vi "Main.vi"() -> ()   [LabVIEW 2021]
panel:
  in  "Numeric":u64 format="%x"
  out "substring":string
  in  "dato":string="F039"
  in  "Write":bool
  in  "Read":bool
  in  "stop":bool
  out "CompleteFrame":string
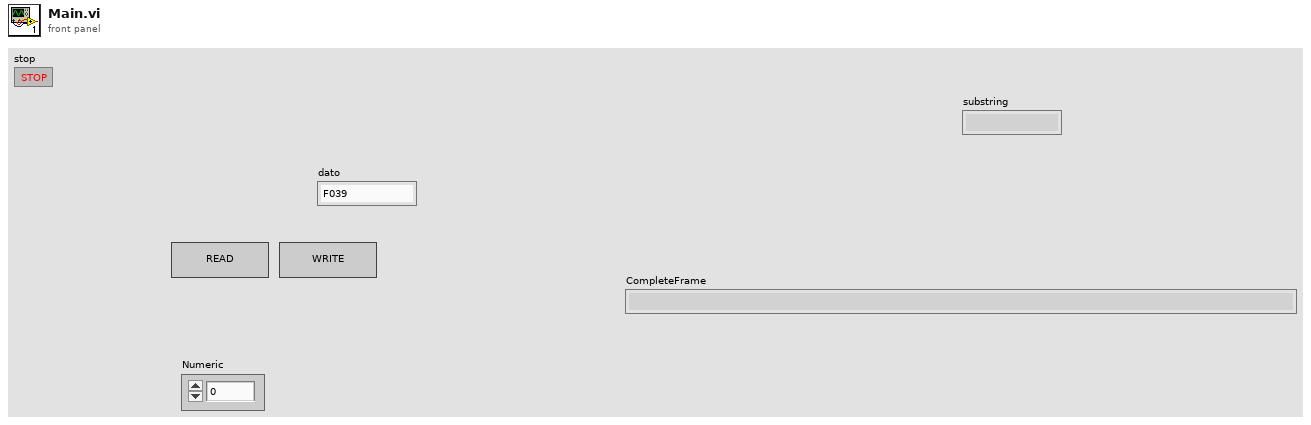
[diagram p1: front panel]
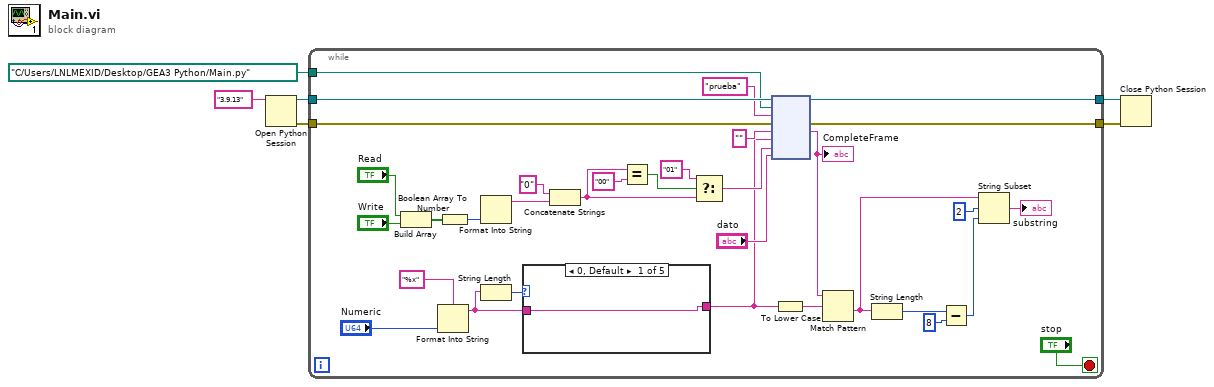
[diagram p0: block diagram]
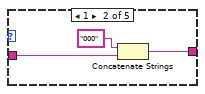
[diagram p2: hidden frame]
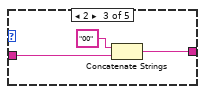
[diagram p3: hidden frame]
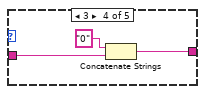
[diagram p4: hidden frame]
diagram:
  n1 = Open Python Session(python version="3.9.13" ("Python version")) -> (session out=w5:refnum<k35>, error out=w4:errorcluster)  [unwired: 2 in]
  n2 = while {
    tunnel: w5 -> [w39]
    tunnel: w4 -> [w38]
    tunnel: [w36] -> w3
    tunnel: [w35] -> w2
    tunnel: path "C:/Users/LNLMEXID/Desktop/GEA3 Python/Main.py" ("module path") -> [w13]
    stop <- "stop" stop-if-true
    n3 = Build Array("Read", "Write") -> (w30:bool[])
    n4 = Format Into String(format string="%x", "Numeric") -> (resulting string=w10:string)  [unwired: 2 in, 1 out]
    n5 = Boolean Array To Number(Boolean array=w30) -> (number=w28:u32)
    n6 = Format Into String(w28) -> (resulting string=w26:string)  [unwired: 3 in, 1 out]
    n7 = String Length(string=w10) -> (length=w12:i32)
    n8 = case shown="0, Default" w12 {
      tunnel: w10 -> [w40 w42 w45 w48 w50]
      tunnel: [w40 w41 w44 w47 w50] -> w8
      frame 0, Default {
      }
      frame 1 {
        n9 = Concatenate Strings("000" ("string"), w42) -> (w41:string)
      }
      frame 2 {
        n10 = Concatenate Strings("00" ("string"), w45) -> (w44:string)
      }
      frame 3 {
        n11 = Concatenate Strings("0" ("string"), w48) -> (w47:string)
      }
      frame 4 {
      }
    }
    n12 = Concatenate Strings("0" ("string"), w26) -> (w22:string)
    n13 = Equal?(x=w22, y="00") -> (x = y?=w24:bool)
    n14 = Select(t="01", s=w24, f=w22) -> (s? t:f=w21:string)
    n15 = node(w39, w13, "prueba" ("function name"), w38, "" ("data_hex"), w8, w21, "dato") -> (w36:refnum<k35>, w35:errorcluster, w20:string)  [unwired: 3 in, 2 out]
    "CompleteFrame" <- w20
    n16 = To Lower Case(string=w8) -> (all lower case string=w7:string)
    n17 = Match Pattern(string=w20, regular expression=w7) -> (after substring=w16:string)  [unwired: 1 in, 3 out]
    n18 = String Length(string=w16) -> (length=w19:i32)
    n19 = Subtract(x=w19, y=8) -> (x-y=w17:i32)
    n20 = String Subset(string=w16, offset (0)=2, length (rest)=w17) -> (substring=→"substring":string)
  }
  n21 = Close Python Session(session in=w3, error in=w2) -> ()  [unwired: 1 out]
